vi "buffer_append.vi"(11 "read buffer":string) -> (0 "Received?":bool, 1 "Alt":string[](array[string]), 2 "Lng":string[](array[string]), 3 "Lat":string[](array[string]), 4 "GPS Valid?":bool)   [LabVIEW 2019]
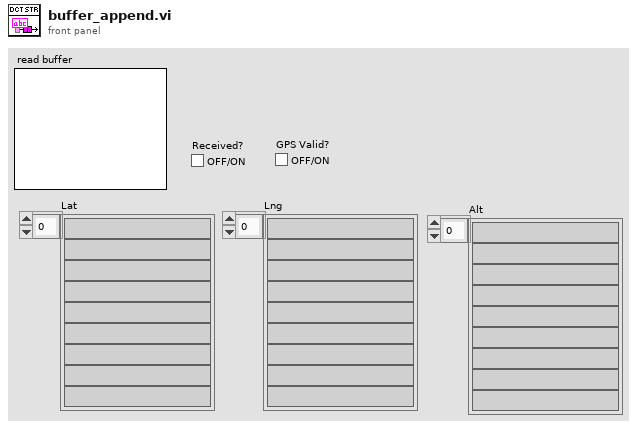
[diagram p1: front panel]
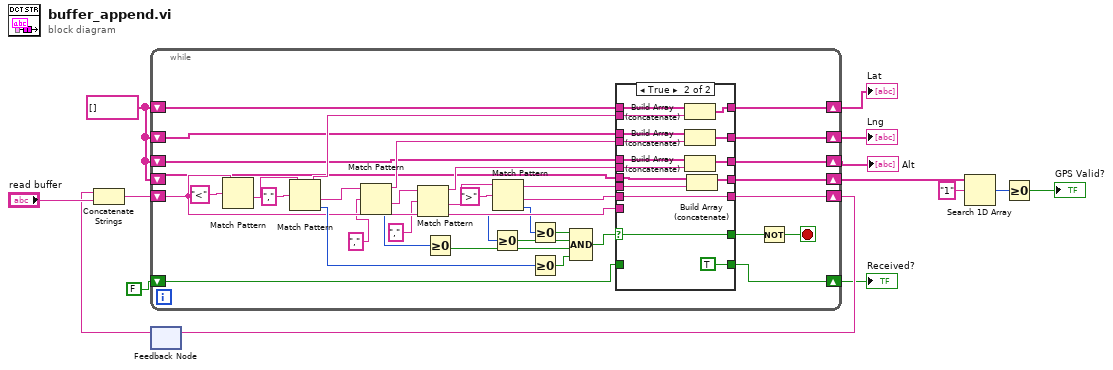
[diagram p0: block diagram]
diagram:
  w7 = string[] []
  n1 = feedback #1() -> (w9:string)  [unwired: 1 in]
  n2 = Concatenate Strings(w9, "read buffer") -> (w11:string)
  n3 = while {
    shift-right: [w38] -> w13
    shift-left: w7 -> [w40]
    shift-right: [w39] -> w14
    shift-left: w7 -> [w41]
    shift-right: [w37] -> w10
    shift-left: w11 -> [w35]
    shift-right: [w34] -> w8
    shift-left: w7 -> [w31]
    shift-right: [w25] -> w6
    shift-left: w7 -> [w23]
    shift-right: [w16] -> w1
    shift-left: FALSE -> [w15]
    stop <- w42 stop-if-true
    n4 = Match Pattern(string=w35, regular expression="<") -> (after substring=w46:string)  [unwired: 1 in, 3 out]
    n5 = Match Pattern(string=w46, regular expression=",") -> (before substring=w47:string, after substring=w33:string, offset past match=w48:i32)  [unwired: 1 in, 1 out]
    n6 = Match Pattern(string=w33, regular expression=",") -> (before substring=w32:string, after substring=w30:string, offset past match=w21:i32)  [unwired: 1 in, 1 out]
    n7 = Match Pattern(string=w30, regular expression=",") -> (before substring=w27:string, after substring=w26:string, offset past match=w20:i32)  [unwired: 1 in, 1 out]
    n8 = Greater Or Equal To 0?(x=w21) -> (x >= 0?=w18:bool)
    n9 = Greater Or Equal To 0?(x=w20) -> (x >= 0?=w19:bool)
    n10 = Match Pattern(string=w26, regular expression=">") -> (before substring=w24:string, after substring=w51:string, offset past match=w22:i32)  [unwired: 1 in, 1 out]
    n11 = Greater Or Equal To 0?(x=w22) -> (x >= 0?=w49:bool)
    n12 = Greater Or Equal To 0?(x=w48) -> (x >= 0?=w17:bool)
    n13 = Compound Arithmetic op=AND(w49, w19, w18, w17) -> (w50:bool)
    n14 = case shown="True" w50 {
      selector: w50 -> [w58 w67]
      tunnel: w47 -> [_ w70]
      tunnel: w27 -> [_ w62]
      tunnel: [w54 w73] -> w37
      tunnel: [w58 w67] -> w36
      tunnel: w51 -> [_ w73]
      tunnel: w41 -> [w56 w72]
      tunnel: w40 -> [w57 w71]
      tunnel: [w56 w69] -> w39
      tunnel: [w57 w68] -> w38
      tunnel: [w55 TRUE] -> w16
      tunnel: w15 -> [w55 _]
      tunnel: w35 -> [w54 _]
      tunnel: [w53 w65] -> w34
      tunnel: w32 -> [_ w63]
      tunnel: w31 -> [w53 w64]
      tunnel: [w52 w61] -> w25
      tunnel: w24 -> [_ w60]
      tunnel: w23 -> [w52 w59]
      frame False {
      }
      frame True {
        n15 = Build Array (concatenate)(w71, w70) -> (w68:string[])
        n16 = Build Array (concatenate)(w72, w63) -> (w69:string[])
        n17 = Build Array (concatenate)(w64, w62) -> (w65:string[])
        n18 = Build Array (concatenate)(w59, w60) -> (w61:string[])
      }
    }
    n19 = Not(x=w36) -> (.not. x?=w42:bool)
  }
  "Lng" <- w14
  "Lat" <- w13
  "Received?" <- w1
  "Alt" <- w8
  n20 = feedback-in #1(w10) -> ()
  n21 = Search 1D Array(1D array=w6, element="1") -> (index of element=w4:i32)  [unwired: 1 in]
  n22 = Greater Or Equal To 0?(x=w4) -> (x >= 0?=→"GPS Valid?":bool)
